vi "ni568x Calibrating CW Test Signal.vi"() -> ()   [LabVIEW 2017]
doc: "This example shows how to make measurements using NI-568x."
uses:
  <instrlib>/ni568x/ni568x.llb/ni568x Initialize - IVI.vi
  <instrlib>/ni568x/ni568x.llb/ni568x Read.vi
panel:
  in  "Resource Name":refnum<k15>
  out "Error Out":errorcluster
  in  "Units":i32(ring)=1 caption="measurement units (dBm)" items=["dBm"=1, "Watts"=4, "mWatts"=1001, "uWatts"=1002]
  out "Reading":dbl
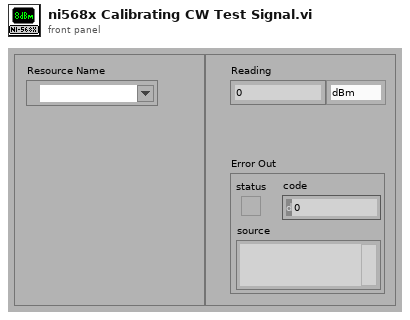
[diagram p1: front panel]
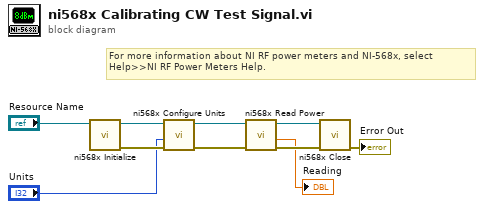
[diagram p0: block diagram]
diagram:
  # "For more information about NI RF power meters and NI-568x, select Help>>NI RF Power Meters Help."
  n1 = call-poly <instrlib>:"ni568x Initialize.vi"("resource name"="Resource Name") -> ("error out"=w5:errorcluster, "instrument handle"=w10:refnum<k15>)  [unwired: 9 in]
  n2 = call <instrlib>:"ni568x Configure Units.vi"("error in"=w5, "units"="Units", "instrument handle"=w10) -> ("error out"=w4:errorcluster, "instrument handle out"=w6:refnum<k15>)  [unwired: 7 in]
  n3 = call-poly <instrlib>:"ni568x Read Power.vi"("error in"=w4, "instrument handle"=w6) -> ("error out"=w8:errorcluster, "power"=→"Reading":dbl, "instrument handle out"=w9:refnum<k15>)  [unwired: 7 in]
  n4 = call <instrlib>:"ni568x Close.vi"("error in"=w8, "instrument handle"=w9) -> ("error out"=→"Error Out":errorcluster)  [unwired: 9 in]
